vi "AlliGator Channel Arithmetic Computation.vi"(8 "Error In":errorcluster, 10 "Channel Arithmetic Action Parameters":T1, 11 "AlliGator IV DVR in":refnum<data-value>) -> (0 "Error Out":errorcluster, 1 "Message":string, 3 "AlliGator IV DVR out":refnum<data-value>)   [LabVIEW 2021, in "AlliGator Dual-Channel Datasets.lvlib"]
doc: "If selected, computes the arithmetic combination of ING & G2 channel and stores it nito the Dataset 1 structure.\n\nIf no arithmetic operation is selected, the G2 channel is in Dataset 1 structure, INT in Dataset 2 structure."
uses:
  AlliGator Dual-Channel Datasets.lvlib
  AlliGator Internal Variables v2.ctl
  <vilib>/vision/Image Controls.llb/IMAQ Image.ctl
  AlliGator Gate Image Set.ctl
  AlliGator FLI Dataset Type.ctl
  AlliGator Data Series Type.ctl
  AlliGator Dataset Channel.ctl
  AlliGator Gate Arithmetic.ctl
  AlliGator Displayed Image.ctl
  Image/Named ROI Description.ctl
  AlliGator Decay Metadata v3.ctl
  AlliGator Decay Background Subtraction Info.ctl
  AlliGator Baseline Subtraction Method.ctl
  Graphs/XY Graph/XY Graph Plot Shift Parameters.ctl
  Graphs/XY Graph/XY Graph Plot Shift Method.ctl
  AlliGator Decay Extrapolation Parameters.ctl
  Phasor/Calibration Phasor (m, phi).ctl
  Phasor/Phasor Reference Series.ctl
  Phasor/Phasor Calibration Map v2.ctl
  Phasor/Phasor (g, s).ctl
  AlliGator Raw Phasor Plot Data v4.ctl
  Phasor/Phasor Standard Deviation Options.ctl
  AlliGator Phasor Multi-Harmonic Data.ctl
  Phasor/Phasor Harmonic Data.ctl
  AlliGator Decay Fit Options & Parameters v2.ctl
  Fits/IRF(X)PSED/Decay Fit Options v2.ctl
  Fits/Decay Convolution/Decay Model.ctl
  Fits/Residual Type.ctl
  Fits/IRF(X)PSED/Fit Weights Type.ctl
  Fits/Non-linear Fitting Method v2.ctl
  Fits/Fit Calculation Method.ctl
  Fits/Non-linear Fitting Algorithm.ctl
  AlliGator Decay Fit Parameter Constraints 2.ctl
  Fits/IRF(X)PSED/Decay Fit Parameters In List.ctl
  Fits/IRF(X)PSED/MLE Baseline Offset Type.ctl
  AlliGator Decay Preprocessing Parameters.ctl
  Fits/IRF(X)PSED/Decay Fit Parameters & Derived Quantities List.ctl
  AlliGator Channel Arithmetic Action Parameters.ctl
  AlliGator Settings List.ctl
  Variant/Variant to Data/Variant to [String].vi
  AlliGator Settings.lvlib
  Variant/Variant to Data/Variant to Data.lvlib
  AlliGator Source Image.lvlib
  Phasor/Phasor.lvlib
  Image/Image.lvlib
  AlliGator Decay Preprocessing.lvlib
  Graphs/XY Graph/XY Graph Add-Ons.lvlib
  AlliGator Phasor Graph.lvlib
  AlliGator Files.lvlib
  AlliGator Internal Variables.lvlib
  AlliGator Phasor Plot.lvlib
  Fits/Fits.lvlib
  AlliGator Decay Fit.lvlib
  AlliGator Decay Fit Parameter Map.lvlib
panel:
  # "see the AlliGator License on the block diagram (Ctrl+E or Window:Show Block Diagram)"
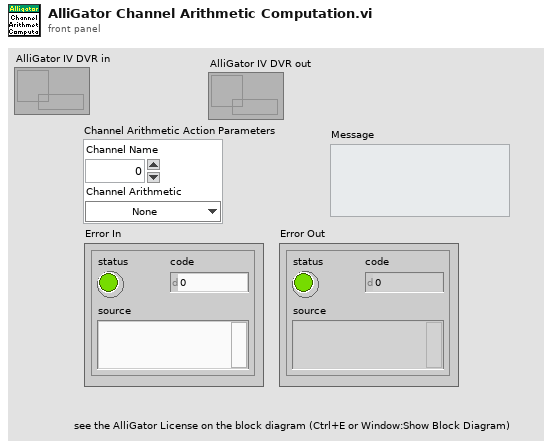
[diagram p1: front panel]
types:
  T1 = typedef "AlliGator Dual-Channel Datasets.lvlib/AlliGator Channel Arithmetic Action Parameters.ctl" = cluster{"Channel Name":u16, "Channel Arithmetic":T2}
  T2 = typedef "AlliGator Settings.lvlib/AlliGator Gate Arithmetic.ctl" = enum16{"None", "INT-G2", "G2/INT*<INT>", "(1 - G2/INT)*<INT>"}
  T3 = typedef "AlliGator Settings.lvlib/AlliGator Settings List.ctl" = enum16{"GUI:Visible Settings Tab", "GUI:Last Run Version", "Source Image:Use Image Histogram for Contrast", "Source Image:Low Count Pixels Rejection Options", "Source Image:High Count Pixels Rejection Options", "Source Image:Use Image Brightness", "Source Image:Blend Overlay with Image Background", "Source Image:Use Fixed ROI Diameter", "Source Image:ROI Diameter", "Source Image:ROI Center Color", "Source Image:Peak Threshold", "Source Image:Intensity Threshold", "Source Image:Image Binning Options", "Source Image:Image Smoothing Options", "Source Image:Image Histogram Active", "Source Image:Invert Binary Mask", "Source Image:Hot Pixel Removal", "Source Image:Overlay Analyzed ROI Center", "Source Image:Auto-Adjust Contrast", "Source Image:Histogram Lower Percentile", "Source Image:Histogram Upper Percentile", "Source Image:Save Source Image", "Source Image:Scale Bar Options", "Source Image:Image Resolution (Pixel Size)", "Source Image:Flatfield Correction", "Source Image:Show Dead Left Columns Correction", "Source Image:Dead Left Columns Correction", "Source Image:Image Pre-Processing Operations Order", "Data Information:Gate Width", "Data Information:Nanotime Gate Separation", "Data Information:Macrotime Gate Separation", "Data Information:Gate Step", "Data Information:# Gates", "Data Information:Gate Image Exposure", "Data Information:Gate Image Integration", "Data Information:Gates to Skip", "Data Information:Gates to Keep", "Data Information:Define Gates to", "Data Information:Channel Name", "Data Information:Available Channel Names", "Data Information:Channel Arithmetic", "Data Information:Background File Subtraction", "Data Information:Background File", "Data Information:Background Scaling Factor", "Data Information:Background Pile-up Correction", "Data Information:Background Pixel Well Capacity", "Data Information:Laser Period", "Data Information:SYNC Period", "Data Information:Pile-up Correction", "Data Information:Pixel Well Capacity", "Data Information:Dataset Scaling Factor", "Fluorescence Decay_Decay Pre-Processing:Reverse Gates", "Fluorescence Decay_Decay Pre-Processing:Verbose Decay Pre-Processing", "Fluorescence Decay_Decay Pre-Processing:Use Decay Pre-Processing", "Fluorescence Decay_Decay Pre-Processing:Background Subtraction", "Fluorescence Decay_Decay Pre-Processing:Background Definition Range", "Fluorescence Decay_Decay Pre-Processing:Baseline Subtraction Method", "Fluorescence Decay_Decay Pre-Processing:Decay Pre-Processing Operations Order", "Fluorescence Decay_Decay Pre-Processing:Smoothing Parameter", "Fluorescence Decay_Decay Pre-Processing:Shift Decay", "Fluorescence Decay_Decay Pre-Processing:Decay Shift Parameters", "Fluorescence Decay_Decay Pre-Processing:Fold Decay", "Fluorescence Decay_Decay Pre-Processing:# Folds", "Fluorescence Decay_Decay Pre-Processing:1-Normalize Decay", "Fluorescence Decay_Decay Pre-Processing:[0-1]-Normalize Decay", "Fluorescence Decay_Decay Pre-Processing:Smoothen Decay", "Fluorescence Decay_Decay Pre-Processing:Extrapolate Decay", "Fluorescence Decay_Decay Pre-Processing:Use Periodicity", "Fluorescence Decay_Decay Pre-Processing:Use Cursors", "Fluorescence Decay_Decay Pre-Processing:Tail Fraction", "Fluorescence Decay_Decay Pre-Processing:Head Fraction", "Fluorescence Decay_Decay Pre-Processing:Additional Points", "Fluorescence Decay_Decay Pre-Processing:Straighten Decay", "Fluorescence Decay_Decay Pre-Processing:Constant Background", "Fluorescence Decay_Decay Pre-Processing:Pixel-Normalize Decay", "Fluorescence Decay_Advanced Analysis:Extract IRF instead of Decay", "Fluorescence Decay_Advanced Analysis:IRF Extraction Options", "Fluorescence Decay_Advanced Analysis:IRF Optimization Options", "Fluorescence Decay_Advanced Analysis:Square Pulse Options", "Fluorescence Decay_Advanced Analysis:IRF Order", "Fluorescence Decay_Advanced Analysis:IRF Time Constants", "Fluorescence Decay_Advanced Analysis:Wavelet Analysis Options", "Fluorescence Decay_Advanced Analysis:Average Lifetime Options", "Fluorescence Decay_Fit Options:Fit Options", "Fluorescence Decay_Fit Options:Use Legacy Fitting Approach", "Fluorescence Decay_Fit Options:Use Data Information Laser Period", "Fluorescence Decay_Fit Parameters:Displayed Fit Parameters", "Fluorescence Decay_Fit Parameters:Fit Parameter Constraints", "Fluorescence Decay_Fit Parameters:Export Tabulated Results", "Fluorescence Decay_Fit Parameters:MLE Baseline Offset Type", "Fluorescence Decay_Fit Parameters:MLE Baseline Offset", "Fluorescence Decay_Fit Parameters:Guess Parameter Names", "Fluorescence Decay_Fit Parameters:Guess Parameter Values", "Fluorescence Decay_Fit Parameters:Guess Parameters Options", "Fluorescence Decay_Styles:Show Last Decay Only", "Fluorescence Decay_Styles:Decay Graph Color Array", "Fluorescence Decay:Decay Graph Active", "Fluorescence Decay Statistics:Min Peak Value", "Fluorescence Decay Statistics:Reject Low Decay Peak Pixels", "Fluorescence Decay Statistics:Reject High Decay Peak Pixels", "Fluorescence Decay Statistics:Max Peak Value", "Time Traces:Use File Timestamp", "Time Traces:Time Step", "Time Traces:Use Intensity Correction File", "Time Traces:Intensity Correction File", "Phasor Plot:Phasor Plot Smoothing Options", "Phasor Plot:Phasor Plot Size", "Phasor Plot:Phasor Plot Graphics Options", "Phasor Plot:Cumulative Phasor Plot", "Phasor Plot:Use Phasor Brightness", "Phasor Plot:Blend Overlay with Phasor Background", "Phasor Plot:Save Phasor Plot", "Phasor Plot:Show References", "Phasor Plot:Phasor Ratio Decay Range", "Phasor Plot:Exponential Fading", "Phasor Plot:Phasor Ratio Reference Colors", "Phasor Plot:Reference Radius", "Phasor Plot:Show Color Map Vertices", "Phasor Plot:Phasor Plot Active", "Phasor Plot:Phasor Ratio Color Map Type", "Phasor Plot:Phasor Ratio Color Map", "Phasor Plot:Phasor Ratio Display Range", "Phasor Plot:Selected Image ROI(s)", "Phasor Plot:All Image ROIs", "Phasor Plot:Selected Phasor Plot ROI(s)", "Phasor Plot:All Phasor Plot ROIs", "Phasor Plot:Phasor Ratio Color-Coded Quantity", "Phasor Plot:Store Phasor Harmonics", "Phasor Plot:Draw Reference Segment", "Phasor Plot:User-Defined Quantity", "Phasor Graph:Phasor Frequency", "Phasor Graph:Phasor Ratio Type", "Phasor Graph:Pixel-level Phasor Computation", "Phasor Graph:Save Phasor Graph", "Phasor Graph:Phasor Graph Active", "Phasor Graph:Phasor SDV Options", "Phasor Calibration:Use Backup Calibration if needed", "Phasor Graph:Define Shortest Lifetime as", "Phasor Calibration:Backup Calibration Type", "Phasor Calibration:Calibration Type", "Phasor Calibration:Calibration Lifetime", "Phasor Calibration:Calibration Map Algorithm", "Single-Exponential Phasor Locus (SEPL):Gate Parameters", "Single-Exponential Phasor Locus (SEPL):User-defined Gate", "Single-Exponential Phasor Locus (SEPL):User-defined IRF", "Single-Exponential Phasor Locus (SEPL):Phasor Parameters", "Single-Exponential Phasor Locus (SEPL):Decay & IRF Parameters", "Single-Exponential Phasor Locus (SEPL):Display Parameters", "Lifetime Analysis:Decay Analysis Parameters", "Lifetime Analysis:Lifetime Map Active", "Plugins:Python Settings", "Miscellaneous:Verbose Mode", "Miscellaneous:Beep after Script", "Miscellaneous:Saved Image File Format", "Miscellaneous:Exported Gate Image Settings", "Miscellaneous:Include Loading in Timing", "Miscellaneous:Verbose Settings Mode", "Miscellaneous:Histogram Options", "Miscellaneous:Beep on Error", "Miscellaneous:# Logical Processors Used", "Miscellaneous:ROI Description Max Characters", "Miscellaneous:Verbose Error Mode", "Miscellaneous:Transparent Mask Color"}
  T4 = typedef "AlliGator Internal Variables.lvlib/AlliGator Internal Variables v2.ctl" = cluster{"Displayed Image":T5, "White Light Image":T5, "Mask Image":T5, "ROI Mask Image":T5, "Current Dataset Images 1":T6, "Background Dataset Images 1":T6, "Current Dataset Images 2":T6, "Background Dataset Images 2":T6, "Current Dataset Arithmetic Images":T6, "Accumulated Dataset Images 1":T6, "Accumulated Dataset Images 2":T6, "Accumulated Dataset Arithmetic Images":T6, "Phasor Plot Image":T5, "Decay Fit Parameter Map Image":T5, "Single Data Point Path":path, "White Light Image Path":path, "Mask Image Path":path, "Time-Series Folder":path, "[Time-Series Paths]":path[], "Current Dataset":i32, "Single Dataset Type":T7, "Current Folder":string, "AlliGator Data Series Type":T8, "# Datasets":i32, "Dual-Channel Dataset":bool, "Selected Channel Name":string, "Dataset Channel":T9, "Channel Arithmetic":T2, "Dual-Channel Background Dataset":bool, "Background Channel":T9, "Dual-Channel Accumulated Dataset":bool, "Start Time":dbl, "[Time-Series Timestamps]":dbl[], "[Intensity Corrections]":dbl[], "Time Series Script":bool, "Type of Displayed Image":T10, "Gate Image Slide":u16, "# Gates":i32, "ROIs":T11[], "ROI Decay":cluster{"t Array":dbl[], "I Array":dbl[]}, "Valid Decay":bool, "Decay  Metadata":T13, "Reference Decay Plot Name":string, "Reference Decay":cluster{"t Array":dbl[], "I Array":dbl[]}, "Decay Shift Plot":cluster{"Time Stamps":dbl[], "Decay Shifts":dbl[]}, "[Decays Max Values]":sgl[], "[Decays Min Values]":sgl[], "Calibration Phasor":T19, "Calibration Phasor Series":T20, "Phasor Calibration Map":T21, "Calibration Map MD5 Digest":string, "Last Raw Phasor":T22, "Last Calibrated Phasor":T22, "Last Calibrated Phasor SDV":T22, "Phasor Graph:Phasor Plot":cluster{"g Array":dbl[], "s Array":dbl[]}, "Phasor Graph:Phasor SDV Plot":cluster{"g Array":dbl[], "s Array":dbl[]}, "[Phasor Graph:Raw Phasor Plots]":T23[], "Phasor Plot locked to Ref 1":i32, "[Phasor Plot(s) locked to Ref 1]":i32[], "[Phasor Plot(s) locked to Ref 2]":i32[], "[Pixel Phasors]":T22[], "[[Sum Image]]":dbl[][], "[[CSG Phasors]]":csg[][], "[[Valid Pixel?]]":bool[][], "I/m/phi Dataset":cluster{"I/m/phi Dataset?":bool, "Base Frequency":dbl[unit], "Harmonic Orders":u8[]}, "Multi Phasor Plot Data":T25, "Decay Fit Options & Parameters":T27, "Fit Options: Decay Preprocessing Parameters":T38, "Fit Options: Reference Decay":cluster{"t Array":dbl[], "I Array":dbl[]}, "Is Full Image Parameters Map":bool, "Is Single-Pixels Parameters Map":bool, "NLSF Parameters Map X Resolution":i32, "NLSF Parameters Map Y Resolution":i32, "[Single Decay Fit Parameters]":dbl[], "Fit Model":T29, "[[Multiple Decays Fit Parameters]]":dbl[][], "[[Multiple Decays Fit Parameter SDVs]]":dbl[][], "[[IRFs]]":dbl[][], "IRF Array Time Axis":dbl[], "Decay Array Time Axis":dbl[], "[Decay Fit Parameter Names]":T39[], "[[Phasor Ratios]]":dbl[][], "[[Average Lifetimes]]":dbl[][], "Amplitude Weighted Average Lifetime":bool, "[Decay Sum]":dbl[], "[[User-defined Quantities]]":dbl[][], "User-defined Quantity":string}
  T5 = typedef "IMAQ Image.ctl" = refnum<image>
  T6 = typedef "AlliGator Internal Variables.lvlib/AlliGator Gate Image Set.ctl" = cluster{"SGL Image Max":T5, "SGL Image Sum":T5, "SGL Gate Images":T5[], "SGL Image Min":T5}
  T7 = typedef "AlliGator Files.lvlib/AlliGator FLI Dataset Type.ctl" = enum16{"HDF5 FLI Dataset", "Gate Image Folder", ".sdt FLI Dataset (Becker & Hickl)", ".ptu FLI Dataset (PicoQuant)", "SS1 FLI Dataset", "SS2 FLI Dataset", "I/m/phi Dataset", ".bin FLI Dataset (PicoQuant Binned)", ".bin FLI Dataset (Piccolo Binned)"}
  T8 = typedef "AlliGator Files.lvlib/AlliGator Data Series Type.ctl" = enum16{"Not a Supported Series", "Gate Images Folder Series", "SwissSPAD 2 Dataset Series", "B&H FLI Dataset Series", "PicoQuant PTU FLI Dataset Series", "PicoQuant BIN FLI Dataset Series", "Piccolo hist BIN FLI Dataset Series", "HDF5 FLI Dataset Series"}
  T9 = typedef "AlliGator Dual-Channel Datasets.lvlib/AlliGator Dataset Channel.ctl" = enum16{"G2", "INT"}
  T10 = typedef "AlliGator Source Image.lvlib/AlliGator Displayed Image.ctl" = enum16{"Single Gate", "Sum of All Gates", "Max of All Gates", "Min of All Gates", "-", "White Ligth Image", "Mask Image"}
  T11 = typedef "Image.lvlib/Named ROI Description.ctl" = cluster{"ROI Descriptor":T12, "ROI Name":string, "Overlay Color":u32}
  T12 = typedef "ROI Descriptor" = cluster{"Global Rectangle":i32[], "Contours":cluster{"ID":enum32{"External", "Internal"}, "Type":u32, "Coordinates":i32[]}[]}
  T13 = typedef "AlliGator Phasor Graph.lvlib/AlliGator Decay Metadata v3.ctl" = cluster{"ROI Descriptor":T12, "ROI Center":cluster{"X":i32, "Y":i32}, "Decay Background Subtraction Info":T14, "Decay Reverted":bool, "Decay Smoothened":bool, "Decay Straightened":bool, "Fitted Tau (Decay Straightening)":dbl, "Decay Shift Parameters":T16, "Decay Shifted":bool, "Decay Extrapolated":bool, "Decay Extrapolation Parameters":T18, "Decay Normalized":bool, "Fold Decay":bool, "# Folds":u32}
  T14 = typedef "AlliGator Decay Analysis.lvlib/AlliGator Decay Preprocessing.lvlib/AlliGator Decay Background Subtraction Info.ctl" = cluster{"Laser Period":dbl[unit], "Gate Duration":dbl[unit], "Baseline Subtraction Method":T15, "Background Definition Range":cluster{"Min Gate":dbl[unit], "Max Gate":dbl[unit]}, "Total Intensity w/o Bkgd Subtraction":dbl, "Bkgd-subtracted Intensity (exp)":dbl, "# Data Points":i32, "Background/Gate":dbl, "Fitted Lifetime":dbl[unit], "Bkgd-subtracted Intensity (theo)":dbl}
  T15 = typedef "AlliGator Decay Analysis.lvlib/AlliGator Decay Preprocessing.lvlib/AlliGator Baseline Subtraction Method.ctl" = enum16{"Mean", "Min", "Square Gated Single-Exponential", "File", "Constant"}
  T16 = typedef "XY Graph Add-Ons.lvlib/XY Graph Plot Shift Parameters.ctl" = cluster{"Type":T17, "Shift":dbl[unit], "Threshold":dbl, "Rotate":bool}
  T17 = typedef "XY Graph Add-Ons.lvlib/XY Graph Plot Shift Method.ctl" = enum16{"Default", "CFD", "Threshold", "Cross-Correlation"}
  T18 = typedef "AlliGator Decay Analysis.lvlib/AlliGator Decay Preprocessing.lvlib/AlliGator Decay Extrapolation Parameters.ctl" = cluster{"Additional Points":u32, "Head Fraction":dbl, "Fitted Tau":dbl, "Use Periodicity":bool, "Use Cursors":bool, "Tail Fraction":dbl}
  T19 = typedef "Phasor.lvlib/Calibration Phasor (m, phi).ctl" = cluster{"m":dbl, "phi":dbl, "Phasor Frequency":dbl[unit], "Reference Lifetime":dbl[unit]}
  T20 = typedef "Phasor.lvlib/Phasor Reference Series.ctl" = cluster{"m Array":dbl[], "phi Array":dbl[], "Phasor Frequency":dbl[unit], "Calibration Lifetime":dbl[unit]}
  T21 = typedef "Phasor.lvlib/Phasor Calibration Map v2.ctl" = cluster{"Phasor Frequency":dbl[unit], "Calibration Lifetime":dbl[unit], "ROI Centers":cluster{"X":i32, "Y":i32}[], "ROI Descriptors":T12[], "Map Resolution X":i32, "Map Resolution Y":i32, "z Array":cdb[]}
  T22 = typedef "Phasor.lvlib/Phasor (g, s).ctl" = cluster{"g":dbl, "s":dbl}
  T23 = typedef "AlliGator Phasor Graph.lvlib/AlliGator Raw Phasor Plot Data v4.ctl" = cluster{"Phasor Plot Name":string, "Raw Phasor Plot":T22[], "Phasor Frequency":dbl[unit], "[Decay Metadata]":T13[], "Raw Phasor Plot SDV":T22[], "Phasor SDV Options":T24, "[Calibration Phasor]":T19[]}
  T24 = typedef "Phasor.lvlib/Phasor Standard Deviation Options.ctl" = cluster{"Compute Estimated SDV":bool, "# Replicas":u32, "Use Estimated Average Phasor":bool}
  T25 = typedef "AlliGator Phasor Plot.lvlib/AlliGator Phasor Multi-Harmonic Data.ctl" = cluster{"Base Frequency":dbl[unit], "# Harmonics":u8, "Harmonic Orders":u8[], "Phasor Plot Settings Checksum":u64, "Phasor Harmonic Data Array":T26[]}
  T26 = typedef "Phasor.lvlib/Phasor Harmonic Data.ctl" = cluster{"Phasor Harmonic Name":string, "Phasor Plot Settings Checksum":u64, "Phasor Frequency":dbl[unit], "Base Frequency":dbl[unit], "Harmonic Order":u8, "Phasor Plot Parameters":string, "Phasor Array [[CSG]]":csg[][], "Dataset File Path":path}
  T27 = typedef "AlliGator Decay Fit Parameter Map.lvlib/AlliGator Decay Fit Options & Parameters v2.ctl" = cluster{"SYNC Period":dbl[unit], "Fit Options":T28, "Fit Parameter Constraints":T35[], "MLE Baseline Offset":dbl, "MLE Baseline Offset Type":T37}
  T28 = typedef "Fits.lvlib/Decay Fit Options v2.ctl" = cluster{"Show Fit Residuals":bool, "Fit Model":T29, "Residual Type":T30, "Max Decay Percentile":dbl, "Min Decay Percentile":dbl, "Show Full Decay":bool, "Weights":T31, "Fitting Method":T32, "Compute Parameter Uncertainties":bool, "Periodic Boundaries":bool, "Model Calculation":T33, "Period":dbl[unit], "Termination Criteria":cluster{"Max Iterations":i32, "Max Function Calls":i32, "Max Time":dbl[unit], "Function Tolerance":dbl, "Parameter Tolerance":dbl, "Gradient Tolerance":dbl, "Min Lambda":dbl, "Max Lambda":dbl, "Initial Tick Count":u32}, "Offset Resolution":dbl[unit], "Use Local IRF":bool, "Fitting Algorithm":T34}
  T29 = typedef "Fits.lvlib/Decay Model.ctl" = enum16{"1-Exponential", "2-Exponentials"}
  T30 = typedef "Fits.lvlib/Residual Type.ctl" = enum16{"Standard", "Normalized", "Reduced"}
  T31 = typedef "Fits.lvlib/Fit Weights Type.ctl" = enum16{"Unweighted", "1/Variance", "Best of All"}
  T32 = typedef "Fits.lvlib/Non-linear Fitting Method v2.ctl" = enum16{"Least Square", "Least Absolute Residual", "Bisquare", "MLE", "-", "Best of All"}
  T33 = typedef "Fits.lvlib/Fit Calculation Method.ctl" = enum16{"Simulation", "Convolution", "Integration"}
  T34 = typedef "Fits.lvlib/Non-linear Fitting Algorithm.ctl" = enum16{"Levenberg-Marquardt", "Trust-Region Dogleg"}
  T35 = typedef "AlliGator Decay Analysis.lvlib/AlliGator Decay Fit.lvlib/AlliGator Decay Fit Parameter Constraints 2.ctl" = cluster{"Fit Parameter":T36, "Min Value":dbl, "Max Value":dbl, "Global":bool, "Used":bool}
  T36 = typedef "Fits.lvlib/Decay Fit Parameters In List.ctl" = enum16{"Offset", "Baseline", "A_1", "tau_1", "A_2", "tau_2"}
  T37 = typedef "Fits.lvlib/MLE Baseline Offset Type.ctl" = enum32{"Absolute", "Percentage"}
  T38 = typedef "AlliGator Decay Analysis.lvlib/AlliGator Decay Preprocessing.lvlib/AlliGator Decay Preprocessing Parameters.ctl" = cluster{"Background Subtraction":bool, "Straighten Decay":bool, "Reverse Gates":bool, "1-Normalized Decay":bool, "Smoothen Decay":bool, "Smoothing Parameter":dbl, "Shift Decay":bool, "Decay Shift Parameters":T16, "Extrapolate Decay":bool, "Additional Points":u32, "Head Fraction":dbl, "Pixel-Normalize Decay":bool, "Use Periodicity":bool, "Use Cursors":bool, "Tail Fraction":dbl, "Use Decay Pre-Processing":bool, "Fold Decay":bool, "# Folds":u32, "[0-1]-Normalized Decay":bool}
  T39 = typedef "Fits.lvlib/Decay Fit Parameters & Derived Quantities List.ctl" = enum16{"Offset", "Baseline", "A_1", "tau_1", "A_2", "tau_2", "<tau>_a", "f1_a", "f2_a", "<tau>_i", "f1_i", "f2_i", "-", "R^2", "Chi^2"}
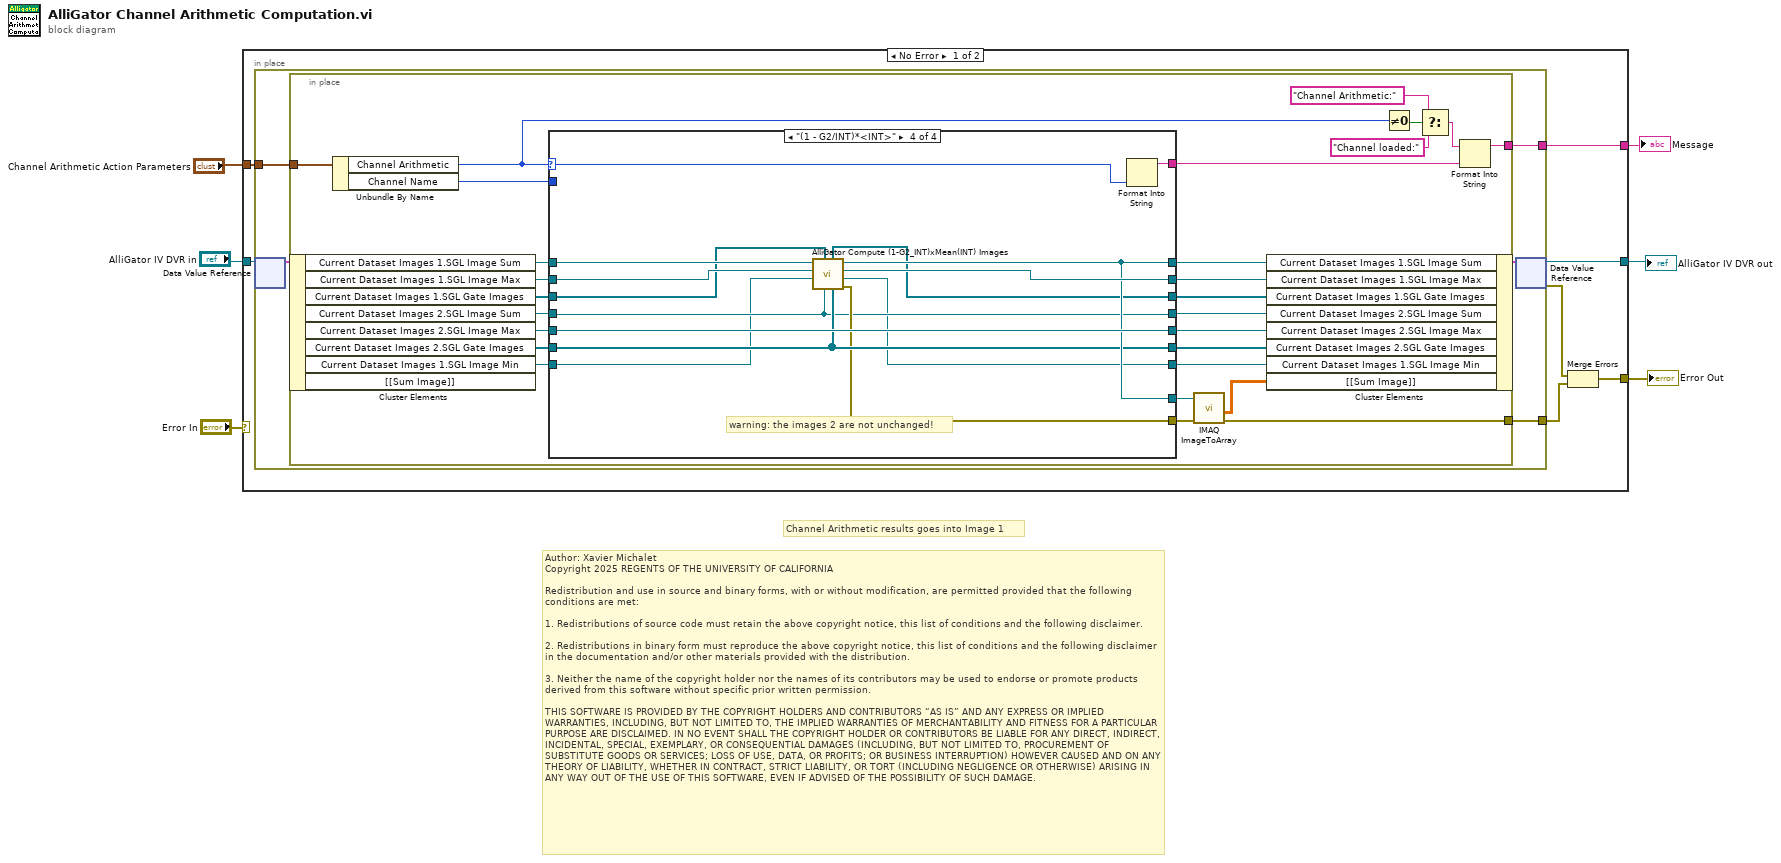
[diagram p0: block diagram]
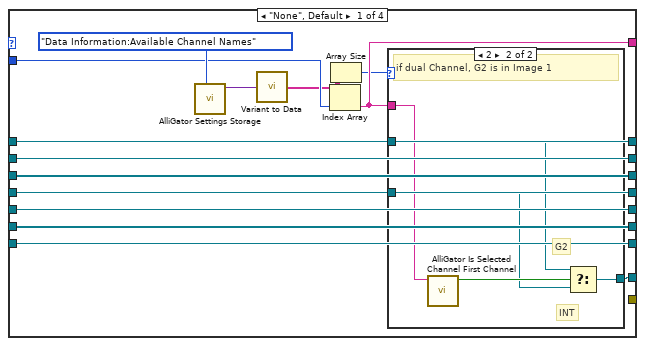
[diagram p2: hidden frame]
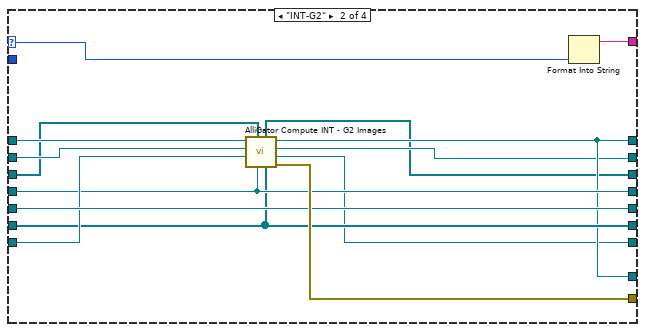
[diagram p4: hidden frame]
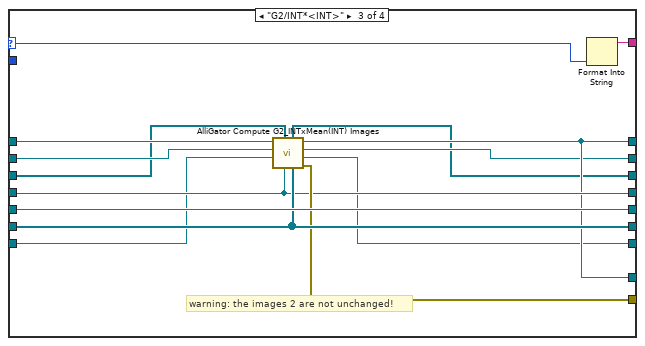
[diagram p5: hidden frame]
diagram:
  # "Author: Xavier Michalet\nCopyright 2025 REGENTS OF THE UNIVERSITY OF CALIFORNIA\n\nRedistribution and use in source and binary forms, with or without modification, are permitted provided that the following conditions are met:\n\n1. Redistributions of source code must retain the above copyright notice, this list of conditions and the following disclaimer.\n\n2. Redistributions in binary form must reproduce the above copyright notice, this list of conditions and the following disclaimer in the documentation and/or other materials provided with the distribution.\n\n3. Neither the name of the copyright holder nor the names of its contributors may be used to endorse or promote products derived from this software without specific prior written permission.\n\nTHIS SOFTWARE IS PROVIDED BY THE COPYRIGHT HOLDERS AND CONTRIBUTORS “AS IS” AND ANY EXPRESS OR IMPLIED WARRANTIES, INCLUDING, BUT NOT LIMITED TO, THE IMPLIED WARRANTIES OF MERCHANTABILITY AND FITNESS FOR A PARTICULAR PURPOSE ARE DISCLAIMED. IN NO EVENT SHALL THE COPYRIGHT HOLDER OR CONTRIBUTORS BE LIABLE FOR ANY DIRECT, INDIRECT, INCIDENTAL, SPECIAL, EXEMPLARY, OR CONSEQUENTIAL DAMAGES (INCLUDING, BUT NOT LIMITED TO, PROCUREMENT OF SUBSTITUTE GOODS OR SERVICES; LOSS OF USE, DATA, OR PROFITS; OR BUSINESS INTERRUPTION) HOWEVER CAUSED AND ON ANY THEORY OF LIABILITY, WHETHER IN CONTRACT, STRICT LIABILITY, OR TORT (INCLUDING NEGLIGENCE OR OTHERWISE) ARISING IN ANY WAY OUT OF THE USE OF THIS SOFTWARE, EVEN IF ADVISED OF THE POSSIBILITY OF SUCH DAMAGE."
  # "Channel Arithmetic results goes into Image 1"
  n1 = case shown="No Error" "Error In" {
    selector: "Error In" -> [_ w109]
    tunnel: [w9 w109] -> w6
    tunnel: "AlliGator IV DVR in" -> [w13 w108]
    tunnel: [w12 w108] -> w4
    tunnel: "Channel Arithmetic Action Parameters" -> [w10 _]
    tunnel: [w7 _] -> w1
    frame No Error {
      n2 = in-place {
        in-place-border: w10 -> [w16]
        in-place-border: [w15] -> w8
        in-place-border: [w14] -> w7
        n3 = in-place-dvr #1(w13) -> (w18:T4)  [unwired: 1 out]
        n4 = in-place {
          in-place-border: w16 -> [w29]
          in-place-border: [w30] -> w15
          in-place-border: [w23] -> w14
          n5 = in-place-cluster #2(w18) -> ("Current Dataset Images 1.SGL Image Sum"=w45:T5, "Current Dataset Images 1.SGL Image Max"=w43:T5, "Current Dataset Images 1.SGL Gate Images"=w41:T5[], "Current Dataset Images 2.SGL Image Sum"=w39:T5, "Current Dataset Images 2.SGL Image Max"=w37:T5, "Current Dataset Images 2.SGL Gate Images"=w35:T5[], "Current Dataset Images 1.SGL Image Min"=w20:T5)  [unwired: 1 out]
          n6 = Unbundle By Name(w29) -> ("Channel Arithmetic"=w25:T2, "Channel Name"=w28:u16)
          n7 = case shown="\"(1 - G2/INT)*<INT>\"" w25 {
            selector: w25 -> [_ w77 w91 w103]
            tunnel: w45 -> [w50 w75 w87 w102]
            tunnel: [w50 w69 w86 w105] -> w44
            tunnel: w43 -> [w59 w74 w85 w101]
            tunnel: [w59 w68 w83 w107] -> w42
            tunnel: w41 -> [w58 w71 w80 w96]
            tunnel: [w58 w67 w81 w95] -> w40
            tunnel: w39 -> [w51 w72 w88 w98]
            tunnel: [w51 w72 w88 w98] -> w38
            tunnel: w37 -> [w57 w76 w93 w106]
            tunnel: [w57 w76 w93 w106] -> w36
            tunnel: w35 -> [w56 w70 w90 w100]
            tunnel: [w56 w70 w90 w100] -> w34
            tunnel: [_ w79 w89 w99] -> w32
            tunnel: [w55 w69 w86 w105] -> w33
            tunnel: w28 -> [w52 _ _ _]
            tunnel: [w49 w78 w92 w104] -> w21
            tunnel: w20 -> [w46 w73 w84 w97]
            tunnel: [w46 w66 w82 w94] -> w19
            frame "None", Default {
              n8 = call "AlliGator Settings Storage.vi"("AlliGator Settings List"=AlliGator_Settings_List."Data Information:Available Channel Names") -> ("Variant Data out"=w53:variant)  [unwired: 9 in, 1 out]
              n9 = call-poly "Variant to Data.vi"("Variant"=w53) -> ("String Array"=w48:string[])  [unwired: 8 in]
              n10 = Index Array(array=w48, index=w52) -> (element=w49:string)
              n11 = Array Size(array=w48) -> (size(s)=w47:i32)
              n12 = case shown="2" w47 {
                tunnel: [w60 w65] -> w55
                tunnel: w51 -> [_ w61]
                tunnel: w50 -> [w60 w62]
                tunnel: w49 -> [_ w64]
                frame 1, Default {
                  # "if single channel, data is Image 1"
                }
                frame 2 {
                  # "INT"
                  # "G2"
                  # "if dual Channel, G2 is in Image 1"
                  n13 = call "AlliGator Is Selected Channel First Channel.vi"("Selected Channel Name"=w64) -> ("First channel?"=w63:bool)  [unwired: 10 in]
                  n14 = Select(t=w62, s=w63, f=w61) -> (s? t:f=w65:T5)
                }
              }
            }
            frame "INT-G2" {
              n15 = call "AlliGator Compute INT - G2 Images.vi"("INT Images"=w70, "Sum(INT)"=w72, "G2 Images"=w71, "Min(G2)"=w73, "Max(G2)"=w74, "Sum(G2)"=w75) -> ("error out"=w79:errorcluster, "Min(INT - G2)"=w66:T5, "Max(INT - G2)"=w68:T5, "Sum(INT - G2)"=w69:T5, "INT - G2"=w67:T5[])  [unwired: 1 in]
              n16 = Format Into String(w77) -> (resulting string=w78:string)  [unwired: 3 in, 1 out]
            }
            frame "G2/INT*<INT>" {
              # "warning: the images 2 are not unchanged!"
              n17 = call "AlliGator Compute G2_INTxMean(INT) Images.vi"("INT Images"=w90, "Sum(INT)"=w88, "G2 Images"=w80, "Min(G2)"=w84, "Max(G2)"=w85, "Sum(G2)"=w87) -> ("Error Out"=w89:errorcluster, "Min(G2/INT*<INT>)"=w82:T5, "Max(G2/INT*<INT>)"=w83:T5, "Sum(G2/INT*<INT>)"=w86:T5, "G2/INT*<INT> Images"=w81:T5[])  [unwired: 1 in]
              n18 = Format Into String(w91) -> (resulting string=w92:string)  [unwired: 3 in, 1 out]
            }
            frame "(1 - G2/INT)*<INT>" {
              # "warning: the images 2 are not unchanged!"
              n19 = call "AlliGator Compute (1-G2_INT)xMean(INT) Images.vi"("INT Images"=w100, "Sum(INT)"=w98, "G2 Images"=w96, "Min(G2)"=w97, "Max(G2)"=w101, "Sum(G2)"=w102) -> ("Error Out"=w99:errorcluster, "Min((1-G2/INT)*<INT>)"=w94:T5, "Max((1-G2/INT)*<INT>)"=w107:T5, "Sum((1-G2/INT)*<INT>)"=w105:T5, "(1-G2/INT)*<INT> Images"=w95:T5[])  [unwired: 1 in]
              n20 = Format Into String(w103) -> (resulting string=w104:string)  [unwired: 3 in, 1 out]
            }
          }
          n21 = call "IMAQ ImageToArray"("error in (no error)"=w32, "Image"=w33) -> ("Image Pixels (Float)"=w31:sgl[][], "error out"=w30:errorcluster)  [unwired: 2 in, 3 out]
          n22 = in-place-cluster #2("Current Dataset Images 1.SGL Image Sum"=w44, "Current Dataset Images 1.SGL Image Max"=w42, "Current Dataset Images 1.SGL Gate Images"=w40, "Current Dataset Images 2.SGL Image Sum"=w38, "Current Dataset Images 2.SGL Image Max"=w36, "Current Dataset Images 2.SGL Gate Images"=w34, "Current Dataset Images 1.SGL Image Min"=w19, "[[Sum Image]]"=w31) -> (w17:T4)
          n23 = Not Equal To 0?(x=w25) -> (x != 0?=w26:bool)
          n24 = Select(t="Channel Arithmetic:" ("Message"), s=w26, f="Channel loaded:" ("Message")) -> (s? t:f=w22:string)
          n25 = Format Into String(initial string=w22, w21) -> (resulting string=w23:string)  [unwired: 2 in, 1 out]
        }
        n26 = in-place-dvr #1(w17) -> (w12:refnum<data-value>, w11:errorcluster)
      }
      n27 = Merge Errors(w11, w8) -> (w9:errorcluster)
    }
    frame Error {
    }
  }
  "Error Out" <- w6
  "AlliGator IV DVR out" <- w4
  "Message" <- w1
